vi "Verify Cal Information.vi"(6 "교정절차 목록 List":refnum<vi>, 7 "Message":string, 8 "error in (no error)":errorcluster caption="에러 입력(에러 없음)", 10 "교정환경":T1, 11 "교정정보 in":T2) -> (0 "error out":errorcluster caption="에러 출력", 1 "절차생성?":bool, 2 "OK?":bool, 3 "파일명":string)   [LabVIEW 2020]
uses:
  Controls/Clst_Cal Info Global.ctl
  Controls/Clst_Atm Info Global.ctl
  <vilib>/Utility/miscctls.llb/LVRowAndColumnUnsignedTypeDef.ctl
  Variables/Global_Cal Info.vi
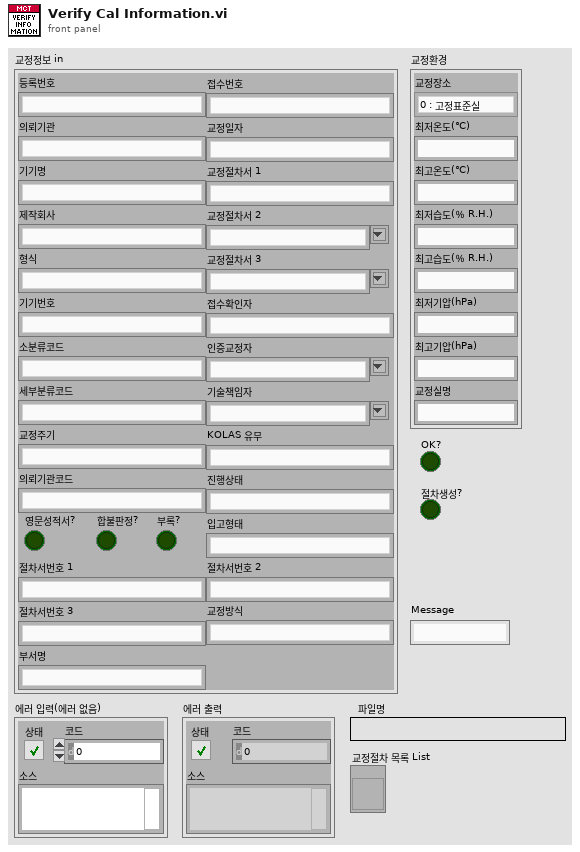
[diagram p1: front panel]
types:
  T1 = typedef "Clst_Atm Info Global.ctl" = cluster{"교정장소":enum16{"0 : 고정표준실", "1 : 현장교정"}, "최저온도(℃)":string, "최고온도(℃)":string, "최저습도(％ R.H.)":string, "최고습도(％ R.H.)":string, "최저기압(hPa)":string, "최고기압(hPa)":string, "교정실명":string}
  T2 = typedef "Clst_Cal Info Global.ctl" = cluster{"등록번호":string, "의뢰기관":string, "기기명":string, "제작회사":string, "형식":string, "기기번호":string, "소분류코드":string, "세부분류코드":string, "교정주기":string, "접수번호":string, "교정일자":string, "교정절차서 1":string, "교정절차서 2":string, "교정절차서 3":string, "접수확인자":string, "인증교정자":string, "기술책임자":string, "KOLAS 유무":string, "진행상태":string, "의뢰기관코드":string, "입고형태":string, "영문성적서?":bool, "합불판정?":bool, "부록?":bool, "절차서번호 1":string, "절차서번호 2":string, "절차서번호 3":string, "교정방식":string, "부서명":string}
  T3 = typedef "LVRowAndColumnUnsignedTypeDef.ctl" = cluster{"Row":u32, "Column":u32}
  T4 = enum32{"invalid app kind", "Development System", "Run Time System", "Student Edition", "Embedded LabVIEW", "Evaluation", "Custom"}
  T5 = cluster{"세부분류코드":string, "형식":string, "옵션":string, "측정기명":string, "EXCEL파일명":string, "TEMP":string}
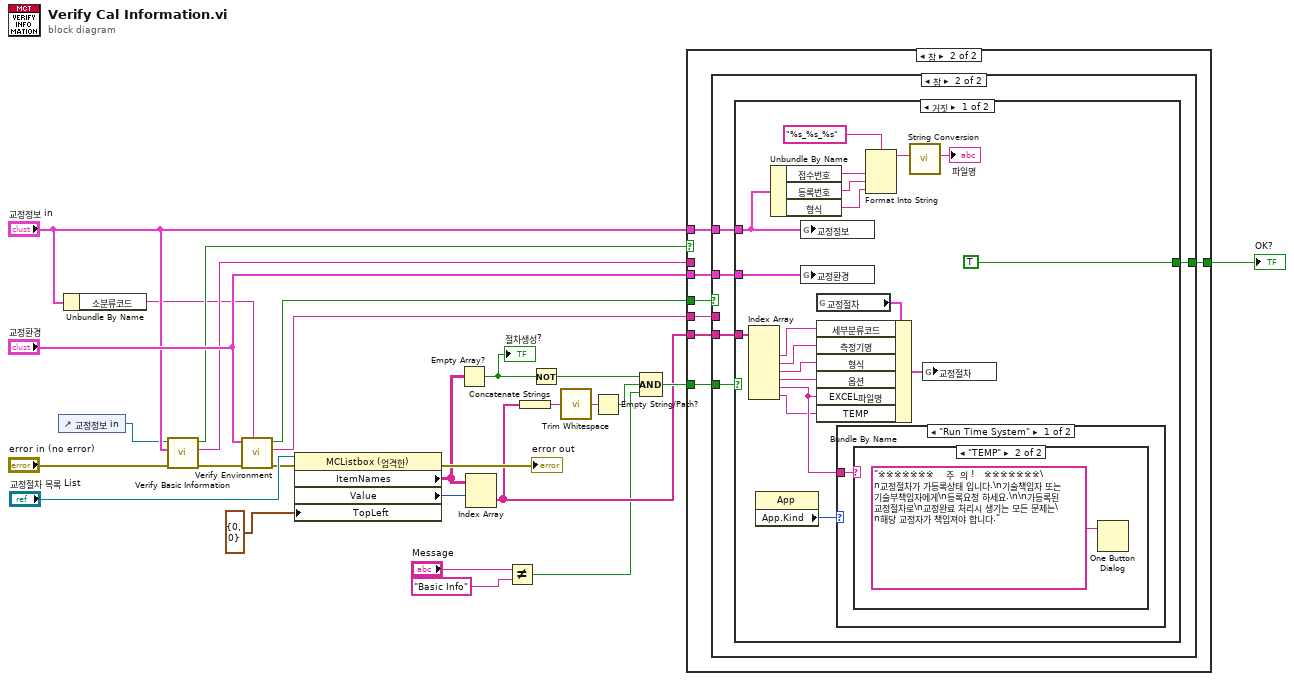
[diagram p0: block diagram]
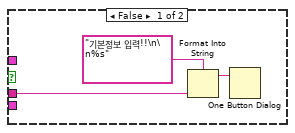
[diagram p2: hidden frame]
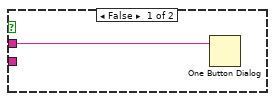
[diagram p3: hidden frame]
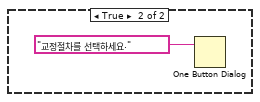
[diagram p6: hidden frame]
diagram:
  n1 = control-ref of="교정정보 in"() -> (w2:refnum<vi>)
  n2 = Unbundle By Name("교정정보 in") -> ("소분류코드"=w17:string)
  n3 = call "Verify Basic Information.vi"("에러 입력(에러 없음)"="error in (no error)", 10:"교정정보 in"="교정정보 in", 11:"교정정보 in"=w2) -> ("에러 출력"=w23:errorcluster, "문자열"=w19:string, "OK?"=w20:bool)  [unwired: 6 in]
  n4 = call "Verify Environment.vi"("소분류코드"=w17, "error in (no error)"=w23, "교정환경"="교정환경") -> ("error out"=w15:errorcluster, "문자열"=w24:string, "OK?"=w25:bool)  [unwired: 6 in]
  n5 = property class="MCListbox (엄격한)"(reference="교정절차 목록 List", error in=w15, "TopLeft"=T3 {"Row"=0, "Column"=0} ("왼쪽 위에 보이는 셀")) -> (error out=→"error out":errorcluster, "ItemNames"=w11:string[][], "Value"=w10:i32)  [unwired: 1 out]
  n6 = Empty Array?(array=w11) -> (empty?=w12:bool)
  "절차생성?" <- w12
  n7 = Index Array(array=w11, index (row)=w10) -> (element=w9:string[])  [unwired: 1 in]
  n8 = Not Equal?(x="Message", y="Basic Info") -> (x != y?=w3:bool)
  n9 = Concatenate Strings(w9) -> (w22:string)
  n10 = Not(x=w12) -> (.not. x?=w7:bool)
  n11 = call <vilib>:"Trim Whitespace.vi"("string"=w22) -> ("trimmed string"=w21:string)  [unwired: 1 in]
  n12 = Empty String/Path?(string/path=w21) -> (empty?=w8:bool)
  n13 = Compound Arithmetic op=AND(w7, w8, w3) -> (w13:bool)
  n14 = case shown="참" w20 {
    tunnel: w19 -> [w30 _]
    tunnel: "교정정보 in" -> [_ w37]
    tunnel: "교정환경" -> [_ w36]
    tunnel: w25 -> [_ w35]
    tunnel: w24 -> [_ w34]
    tunnel: w13 -> [_ w33]
    tunnel: w9 -> [_ w32]
    tunnel: [_ w31] -> w6
    frame False {
      n15 = Format Into String(format string="기본정보 입력!!\n\n%s" ("메시지"), w30) -> (resulting string=w28:string)  [unwired: 2 in, 1 out]
      n16 = One Button Dialog(message=w28) -> ()  [unwired: 1 in, 1 out]
    }
    frame True {
      n17 = case shown="참" w35 {
        tunnel: w37 -> [_ w43]
        tunnel: w36 -> [_ w42]
        tunnel: w34 -> [w38 _]
        tunnel: w33 -> [_ w41]
        tunnel: w32 -> [_ w40]
        tunnel: [_ w39] -> w31
        frame False {
          n18 = One Button Dialog(message=w38) -> ()  [unwired: 1 in, 1 out]
        }
        frame True {
          n19 = case shown="거짓" w41 {
            tunnel: w43 -> [w58 _]
            tunnel: w42 -> [w62 _]
            tunnel: w40 -> [w59 _]
            tunnel: [TRUE _] -> w39
            frame False {
              n20 = Index Array(array=w59) -> (element #2=w50:string, element #3=w47:string, element #4=w49:string, element #5=w48:string, element #6=w46:string, element #7=w44:string)  [unwired: 7 in, 1 out]
              n21 = property class="App"() -> ("App.Kind"=w45:T4)  [unwired: 2 in, 2 out]
              n22 = Unbundle By Name(w58) -> ("접수번호"=w57:string, "등록번호"=w56:string, "형식"=w55:string)
              n23 = global write "Global_Cal Info.vi" "교정정보"(w58) -> ()
              n24 = global write "Global_Cal Info.vi" "교정환경"(w62) -> ()
              n25 = global read "Global_Cal Info.vi" "교정절차"() -> (w61:T5)
              n26 = Bundle By Name(cluster=w61, "세부분류코드"=w50, "측정기명"=w47, "형식"=w49, "옵션"=w48, "EXCEL파일명"=w46, "TEMP"=w44) -> (w60:T5)
              n27 = case shown="\"Run Time System\"" w45 {
                tunnel: w46 -> [w63 _]
                frame "Run Time System" {
                  n28 = case shown="\"TEMP\"" w63 {
                    frame Default {
                    }
                    frame "TEMP" {
                      n29 = One Button Dialog(message="※※※※※※※    주  의 !   ※※※※※※※\n교정절차가 가등록상태 입니다.\n기술책임자 또는 기술부책임자에게\n등록요청 하세요.\n\n가등록된 교정절차로\n교정완료 처리시 생기는 모든 문제는\n해당 교정자가 책임져야 합니다." ("메시지")) -> ()  [unwired: 1 in, 1 out]
                    }
                  }
                }
                frame Default {
                }
              }
              n30 = Format Into String(format string="%s_%s_%s" ("포맷 문자열"), w57, w56, w55) -> (resulting string=w53:string)  [unwired: 2 in, 1 out]
              n31 = call "String Conversion.vi"("문자열 입력"=w53) -> ("변경된 문자열 출력"=→"파일명":string)  [unwired: 10 in]
              n32 = global write "Global_Cal Info.vi" "교정절차"(w60) -> ()
            }
            frame True {
              n33 = One Button Dialog(message="교정절차를 선택하세요." ("메시지")) -> ()  [unwired: 1 in, 1 out]
            }
          }
        }
      }
    }
  }
  "OK?" <- w6
